vi "Select Channels.vi"(8 "error in (no error)":errorcluster, 11 "Node Ptr":u64 format="%.0x") -> (0 "error out":errorcluster)   [LabVIEW 2015, in "J1939 Addon System Explorer.lvlib"]
uses:
  J1939 Addon System Explorer.lvlib
  Shared/SubVIs/Constants.vi
  Protection Support/Source/System Explorer/Protection and Counter Support System Explorer.lvlib
  Shared/J1939 Addon Shared.lvlib
panel:
  in  "Tag":string
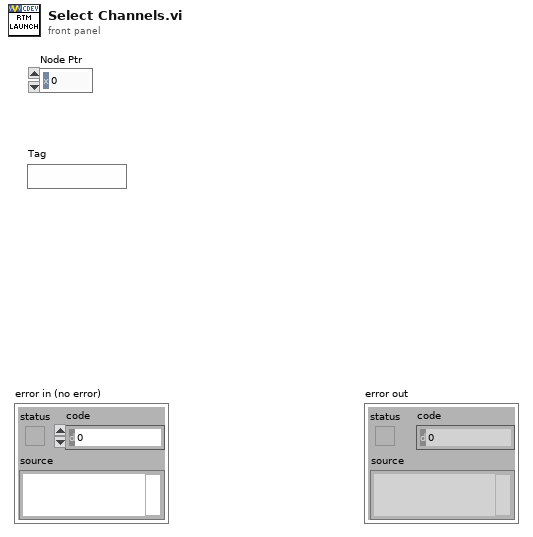
[diagram p1: front panel]
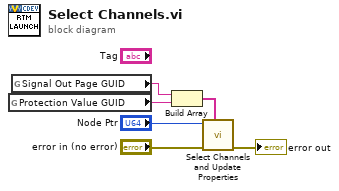
[diagram p0: block diagram]
diagram:
  n1 = global read "Constants.vi" "Protection Value GUID"() -> (w1:string)
  n2 = global read "Constants.vi" "Signal Out Page GUID"() -> (w2:string)
  n3 = Build Array(w2, w1) -> (w3:string[])
  n4 = call "Select Channels and Update Properties.vi"("guids"=w3, "error in (no error)"="error in (no error)", "Node Ptr"="Node Ptr") -> ("error out"=→"error out":errorcluster)  [unwired: 8 in]
